vi "Global R.vi"() -> ()   [LabVIEW 2013]
panel:
  out "R":T1
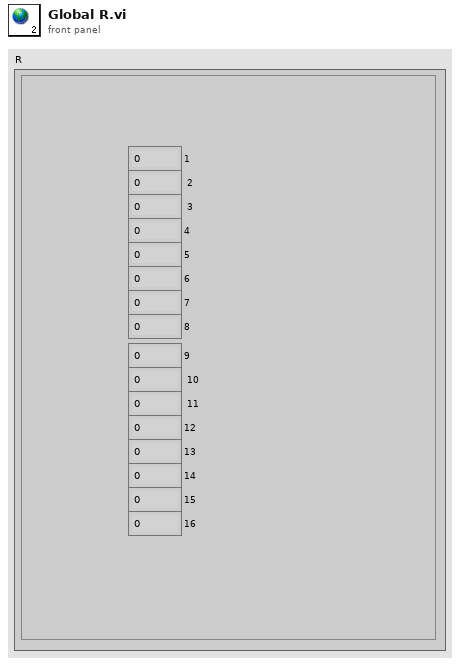
[diagram p1: front panel]
types:
  T1 = cluster{"1":dbl, " 2":dbl, " 3":dbl, "4":dbl, "5":dbl, "6":dbl, "7":dbl, "8":dbl, "9":dbl, " 10":dbl, " 11":dbl, "12":dbl, "13":dbl, "14":dbl, "15":dbl, "16":dbl}
diagram:
